vi "Brewer Palette Dialog v2.vi"() -> (0 "OK?":bool, 1 "Cancelled?":bool, 2 "Interpolate?":bool, 3 "Selected Palette Colors":u32[](array[colorbox]), 5 "Palette Name (# Colors)":string)   [LabVIEW 2021, in "Palette.lvlib"]
doc: "The Palette Colors array returned was chosen by the user while it was displayed vertically.\nIn other words, the top color is in fact color index 0, while the bottom color is in fact the last color in the array.\nTo use this array for a color ramp (or color scale), this array will need to be inverted to obtain the same visual effect."
uses:
  Palette.lvlib
  Utilities/Utilities.lvlib
  Error/Error.lvlib
  <vilib>/IlluminatedG/IG AutoComplete/AutoComplete/AutoComplete.lvlib
panel:
  in  "Matching Palette Names":i32(listbox)
  in  "Search by name":string
  in  "Show Tip Strip":bool
  out "Max  # Colors":i32=3 min=3 max=12 step=1
  in  "About":bool
  in  "Interpolate":bool
  in  "Flip Order":bool
  out "Color Ramp":dbl(ramp)
  in  "Palette List":string(combo)
  in  "Cancel":bool
  in  "OK":bool
  out "Palette Colors":u32[](array[colorbox])
  out "# Palettes":i32=3 min=3 max=12 step=1
  in  "Category":T1(ring)
  in  "photocopy safe":bool
  in  "printer friendly":bool
  in  "colorblind safe":bool
  in  "# Colors":i32=3 min=3 max=15 step=1
  in  "Background":u32(colorbox)=16777226
  # "https://colorbrewer2.org/"
  # "For a visual catalog of Brewer palettes, go to"
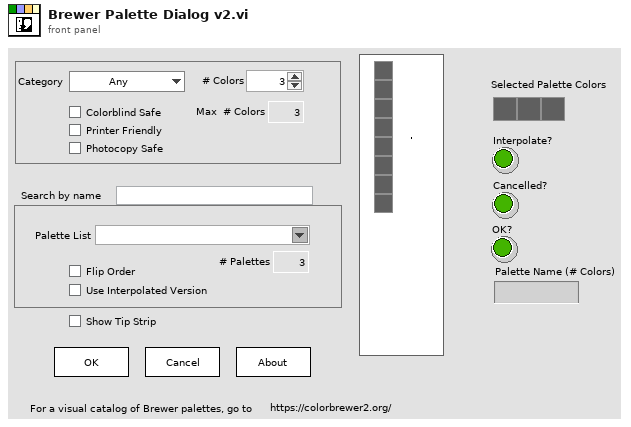
[diagram p1: front panel]
types:
  T1 = enum16{"Any", "Sequential", "Diverging", "Qualitative"}
  T2 = cluster{"Category":enum16{"Any", "Sequential", "Diverging", "Qualitative"}, "photocopy safe":bool, "printer friendly":bool, "colorblind safe":bool, "# Colors":i32, "Flip Order":bool}
  T3 = typedef "Palette.lvlib/Color Brewer Palette.ctl" = cluster{"Color Array":u32[], "Palette Name":string, "Number of Colors":i32, "Palette Category":string, "Color Blind Safe":bool, "Printer Friendly":bool, "Photocopy Safe":bool}
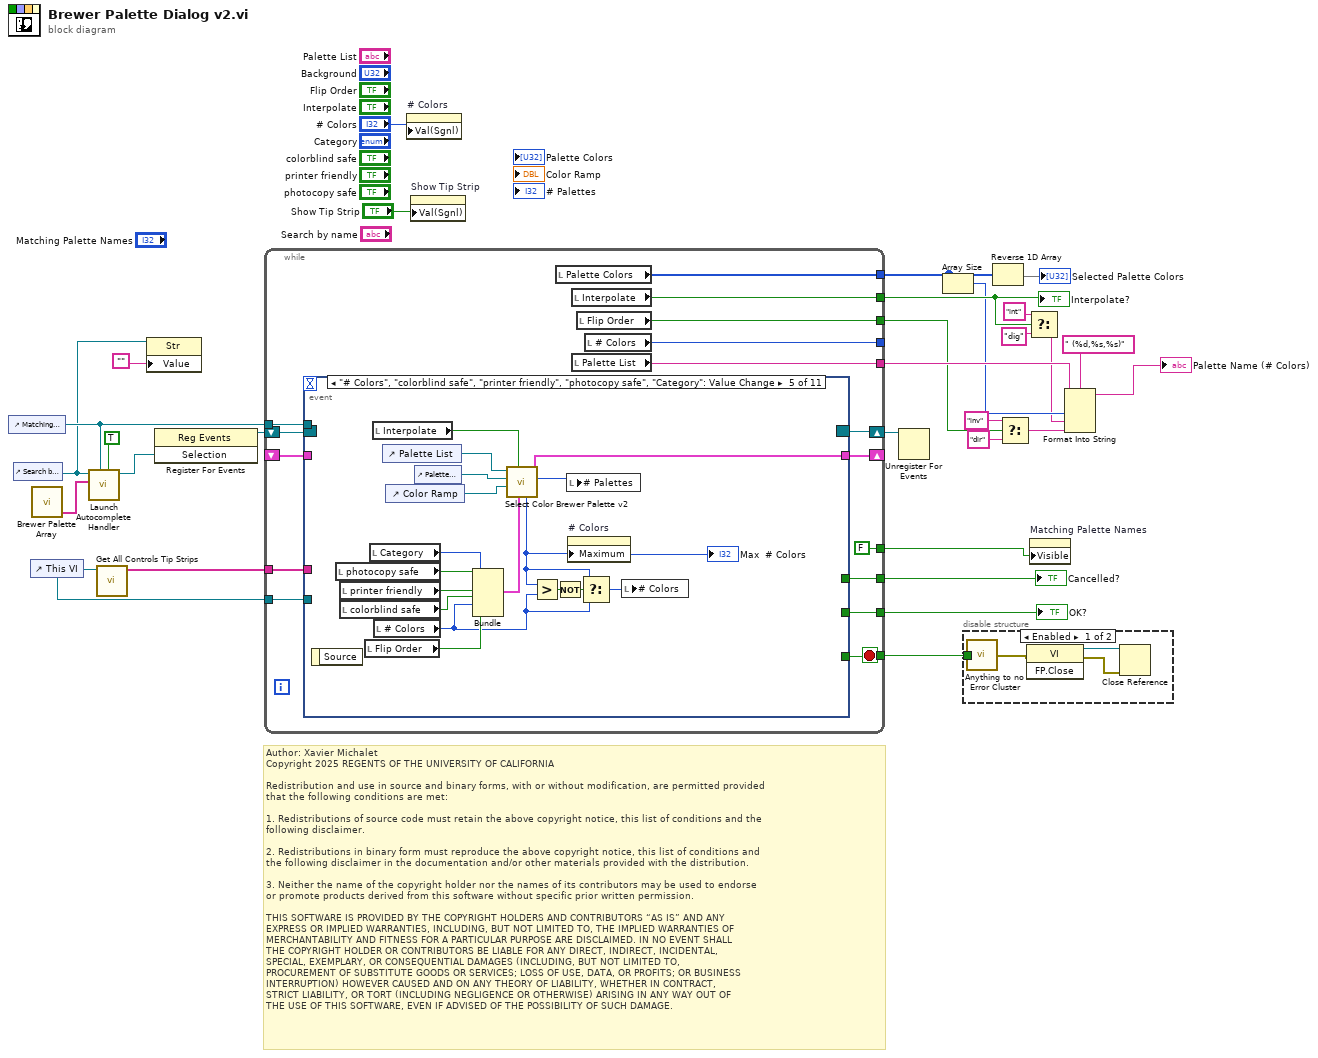
[diagram p0: block diagram]
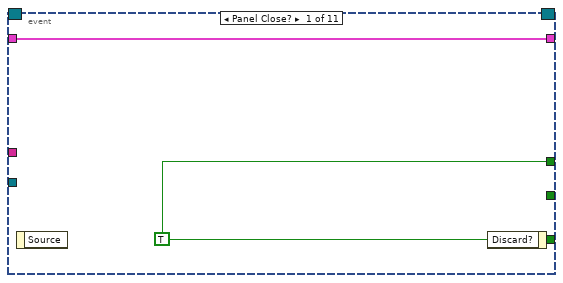
[diagram p3: hidden frame]
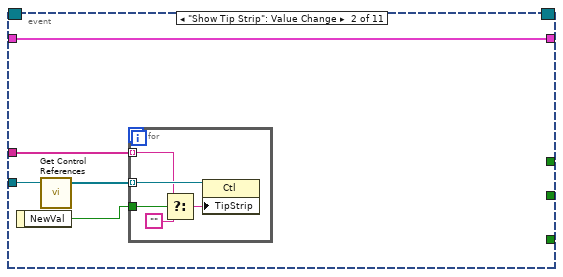
[diagram p4: hidden frame]
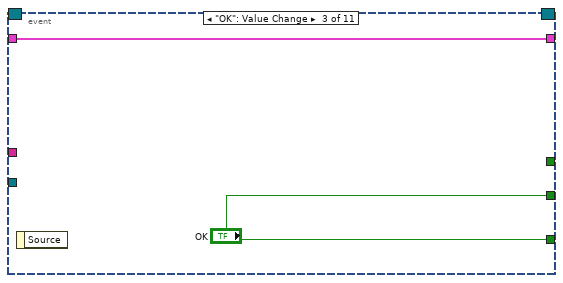
[diagram p5: hidden frame]
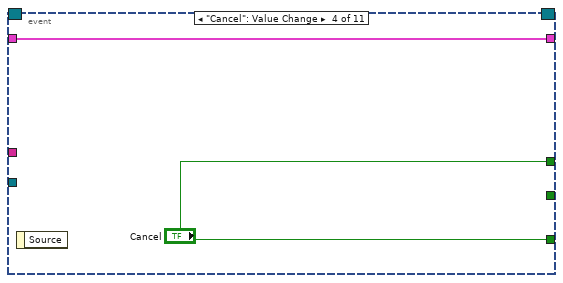
[diagram p6: hidden frame]
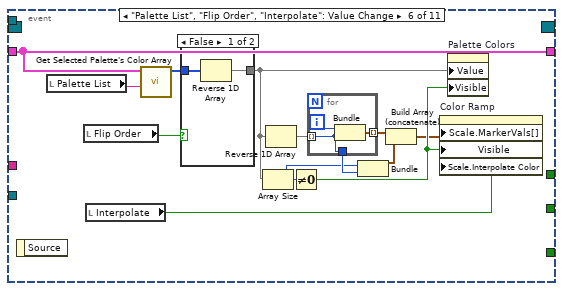
[diagram p7: hidden frame]
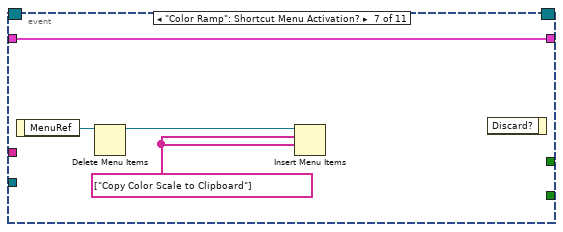
[diagram p9: hidden frame]
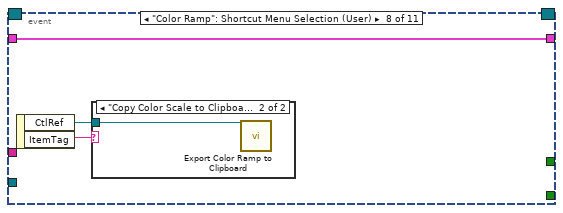
[diagram p10: hidden frame]
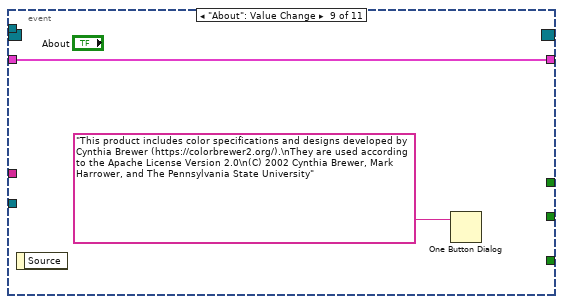
[diagram p12: hidden frame]
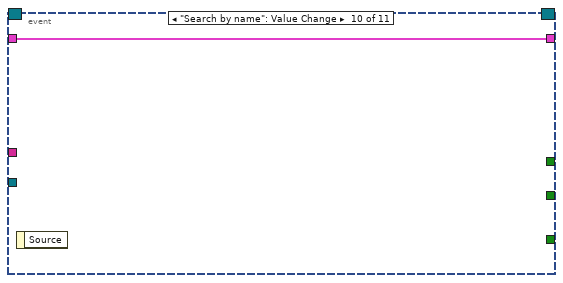
[diagram p13: hidden frame]
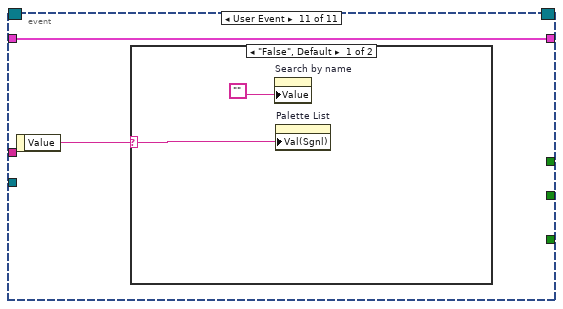
[diagram p14: hidden frame]
diagram:
  # "Author: Xavier Michalet\nCopyright 2025 REGENTS OF THE UNIVERSITY OF CALIFORNIA\n\nRedistribution and use in source and binary forms, with or without modification, are permitted provided\nthat the following conditions are met:\n\n1. Redistributions of source code must retain the above copyright notice, this list of conditions and the\nfollowing disclaimer.\n\n2. Redistributions in binary form must reproduce the above copyright notice, this list of conditions and\nthe following disclaimer in the documentation and/or other materials provided with the distribution.\n\n3. Neither the name of the copyright holder nor the names of its contributors may be used to endorse \nor promote products derived from this software without specific prior written permission.\n\nTHIS SOFTWARE IS PROVIDED BY THE COPYRIGHT HOLDERS AND CONTRIBUTORS “AS IS” AND ANY \nEXPRESS OR IMPLIED WARRANTIES, INCLUDING, BUT NOT LIMITED TO, THE IMPLIED WARRANTIES OF\nMERCHANTABILITY AND FITNESS FOR A PARTICULAR PURPOSE ARE DISCLAIMED. IN NO EVENT SHALL\nTHE COPYRIGHT HOLDER OR CONTRIBUTORS BE LIABLE FOR ANY DIRECT, INDIRECT, INCIDENTAL, \nSPECIAL, EXEMPLARY, OR CONSEQUENTIAL DAMAGES (INCLUDING, BUT NOT LIMITED TO, \nPROCUREMENT OF SUBSTITUTE GOODS OR SERVICES; LOSS OF USE, DATA, OR PROFITS; OR BUSINESS\nINTERRUPTION) HOWEVER CAUSED AND ON ANY THEORY OF LIABILITY, WHETHER IN CONTRACT, \nSTRICT LIABILITY, OR TORT (INCLUDING NEGLIGENCE OR OTHERWISE) ARISING IN ANY WAY OUT OF\nTHE USE OF THIS SOFTWARE, EVEN IF ADVISED OF THE POSSIBILITY OF SUCH DAMAGE."
  n1 = control-ref of="Matching Palette Names"() -> (w5:refnum<vi>)
  n2 = control-ref of="Search by name"() -> (w4:refnum<vi>)
  n3 = control-ref of="This VI"() -> (w11:refnum<vi>)
  n4 = call "Brewer Palette Array.vi"() -> ("Palette List"=w9:string[])  [unwired: 8 in, 1 out]
  n5 = call <vilib>:"Launch Autocomplete Handler.vi"("Autohide ListBox (F)"=TRUE, "ListBox Refnum (Popup)"=w5, "Initial Options (Empty)"=w9, "Str Refnum"=w4) -> ("Selection"=w8:refnum<user-event>)  [unwired: 4 in, 3 out]
  n6 = call "Get All Controls Tip Strips.vi"("VI Ref"=w11) -> ("Controls Tip Strips"=w13:string[])  [unwired: 9 in, 1 out]
  n7 = property class="Str"(reference=w4, "Value"="") -> ()  [unwired: 1 in, 2 out]
  n8 = register-events(w8) -> (reference out=w7:refnum<event-registration>)  [unwired: 2 in, 1 out]
  n9 = while {
    shift-right: [w46] -> _
    shift-left: _ -> [w45]
    tunnel: [w44] -> w30
    tunnel: [w43] -> w29
    tunnel: [w42] -> w27
    tunnel: [w41] -> _
    tunnel: [w40] -> w24
    tunnel: [w39] -> w22
    tunnel: [w38] -> w23
    tunnel: w11 -> [w37]
    tunnel: w13 -> [w36]
    tunnel: [w35] -> w10
    shift-right: [w33] -> w6
    shift-left: w7 -> [w34]
    tunnel: w5 -> [w32]
    tunnel: [FALSE ("Visible")] -> w1
    stop <- w35 stop-if-true
    n10 = event shown="[4] \"# Colors\", \"colorblind safe\", \"printer friendly\", \"photocopy safe\", \"Category\": Value Change" {
      selector: w34 -> [_ _ _ _ _ _ _ _ _ _ _]
      dyn-events: [_ _ _ _ _ _ _ _ _ _ _] -> w33
      timeout: _ -> [_ _ _ _ _ _ _ _ _ _ _]
      tunnel: [w47 _ "OK" "Cancel" _ _ _ _ _ _ _] -> w35
      tunnel: [w48 w53 w59 w61 w73 w92 w102 w105 w108 w109 w111] -> w46
      tunnel: w45 -> [w48 w53 w59 w61 _ w92 w102 w105 w108 w109 w111]
      tunnel: [_ _ "OK" _ _ _ _ _ _ _ _] -> w44
      tunnel: [w47 _ _ "Cancel" _ _ _ _ _ _ _] -> w43
      tunnel: w37 -> [_ w52 _ _ _ _ _ _ _ _ _]
      tunnel: w36 -> [_ w49 _ _ _ _ _ _ _ _ _]
      tunnel: w32 -> [_ _ _ _ _ _ _ _ _ _ _]
      event Panel Close? {
        w47 = TRUE ("Discard?")
        n11 = event-data() -> ()  [unwired: 1 in, 1 out]
        n12 = event-data("Discard?"=w47) -> ()  [unwired: 1 in, 1 out]
      }
      event "Show Tip Strip": Value Change {
        n13 = event-data() -> ("NewVal"=w50:bool)  [unwired: 1 in]
        n14 = call "Get Control References.vi"("VI  Ref"=w52) -> ("Controls[]"=w51:refnum<vi>[])  [unwired: 2 in, 2 out]
        n15 = for {
          tunnel: w51 -> [w58] mode=indexing
          tunnel: w50 -> [w57]
          tunnel: w49 -> [w55] mode=indexing
          n16 = Select(t=w55, s=w57, f="") -> (s? t:f=w56:string)
          n17 = property class="Ctl"(reference=w58, "TipStrip"=w56) -> ()  [unwired: 1 in, 2 out]
        }
      }
      event "OK": Value Change {
        n18 = event-data() -> ()  [unwired: 1 in, 1 out]
      }
      event "Cancel": Value Change {
        n19 = event-data() -> ()  [unwired: 1 in, 1 out]
      }
      event "# Colors", "colorblind safe", "printer friendly", "photocopy safe", "Category": Value Change {
        n20 = event-data() -> ()  [unwired: 1 in, 1 out]
        n21 = local read "photocopy safe"() -> (w78:bool)
        n22 = local read "printer friendly"() -> (w77:bool)
        n23 = local read "colorblind safe"() -> (w76:bool)
        n24 = local read "Flip Order"() -> (w69:bool)
        n25 = local read "Category"() -> (w79:T1)
        n26 = local read "Interpolate"() -> (w63:bool)
        n27 = local read "# Colors"() -> (w67:i32)
        n28 = control-ref of="Palette List"() -> (w72:refnum<vi>)
        n29 = control-ref of="Color Ramp"() -> (w70:refnum<vi>)
        n30 = control-ref of="Palette Colors"() -> (w75:refnum<vi>)
        n31 = Bundle("Category"=w79, "photocopy safe"=w78, "printer friendly"=w77, "colorblind safe"=w76, "# Colors"=w67, "Flip Order"=w69) -> (w71:T2)  [unwired: 1 in]
        n32 = call "Select Color Brewer Palette v2.vi"("User Choices"=w71, "Interpolate"=w63, "Color Ramp Refnum"=w70, "Palette Colors"=w75, "Palette List Refnum"=w72) -> ("# Palettes"=w74:i32, "Available Palettes"=w73:T3[], "Compatible Max # Colors"=w64:i32)  [unwired: 2 in, 2 out]
        "Max  # Colors" <- w64
        n33 = Greater?(x=w64, y=w67) -> (0:w68:bool)
        n34 = Not(x=w68) -> (.not. x?=w65:bool)
        n35 = local write "# Palettes"(w74) -> ()
        n36 = property on="# Colors" class="DigNum (strict)"("Maximum"=w64) -> ()  [unwired: 2 in, 2 out]
        n37 = Select(t=w64, s=w65, f=w67) -> (s? t:f=w66:i32)
        n38 = local write "# Colors"(w66) -> ()
      }
      event "Palette List", "Flip Order", "Interpolate": Value Change {
        n39 = event-data() -> ()  [unwired: 1 in, 1 out]
        n40 = local read "Palette List"() -> (w87:string)
        n41 = local read "Flip Order"() -> (w91:bool)
        n42 = local read "Interpolate"() -> (w84:bool)
        n43 = call "Get Selected Palette's Color Array.vi"("Selected Palette"=w87, "Palette Specifications"=w92) -> ("Palette Colors"=w90:u32[])  [unwired: 8 in, 1 out]
        n44 = case shown="False" w91 {
          tunnel: w90 -> [w97 w98]
          tunnel: [w96 w98] -> w86
          frame False {
            n45 = Reverse 1D Array(array=w97) -> (reversed array=w96:u32[])
          }
          frame True {
          }
        }
        n46 = Array Size(array=w86) -> (size(s)=w80:i32)
        n47 = Reverse 1D Array(array=w86) -> (reversed array=w89:u32[])
        n48 = Not Equal To 0?(x=w80) -> (x != 0?=w85:bool)
        n49 = for {
          tunnel: w89 -> [w93] mode=indexing
          tunnel: [w94] -> w88 mode=indexing
          tunnel: [w93] -> w81
          i -> [w95]
          n50 = Bundle(w95, "Color Box"=w93) -> (w94:cluster{i32, "Color Box":u32})  [unwired: 1 in]
        }
        n51 = Bundle(w80, "Color Box"=w81) -> (w82:cluster{i32, "Color Box":u32})  [unwired: 1 in]
        n52 = Build Array (concatenate)(w88, w82) -> (w83:cluster{i32, "Color Box":u32}[])
        n53 = property on="Color Ramp" class="ColRmp (strict)"("Scale.MarkerVals[]"=w83, "Visible"=w85, "Scale.Interpolate Color"=w84) -> ()  [unwired: 2 in, 2 out]
        n54 = property on="Palette Colors" class="Arr (strict)"("Value"=w86, "Visible"=w85) -> ()  [unwired: 2 in, 2 out]
      }
      event "Color Ramp": Shortcut Menu Activation? {
        w100 = string[] ["Copy Color Scale to Clipboard"] ("item names")
        n55 = event-data() -> ("MenuRef"=w99:refnum<k9>)  [unwired: 1 in]
        n56 = Delete Menu Items(9:w99) -> (3:w101:refnum<k9>)  [unwired: 3 in, 1 out]
        n57 = Insert Menu Items(7:w100, 8:w100, 9:w101) -> ()  [unwired: 3 in, 3 out]
        n58 = event-data() -> ()  [unwired: 2 in, 1 out]
      }
      event "Color Ramp": Shortcut Menu Selection (User) {
        n59 = event-data() -> ("CtlRef"=w103:refnum<vi>, "ItemTag"=w104:string)  [unwired: 1 in]
        n60 = case shown="\"Copy Color Scale to Clipboard\"" w104 {
          tunnel: w103 -> [_ w106]
          frame "", Default {
          }
          frame "Copy Color Scale to Clipboard" {
            n61 = call "Export Color Ramp to Clipboard.vi"("ColorRamp in"=w106) -> ()  [unwired: 11 in]
          }
        }
      }
      event "About": Value Change {
        n62 = event-data() -> ()  [unwired: 1 in, 1 out]
        n63 = One Button Dialog(message="This product includes color specifications and designs developed by Cynthia Brewer (https://colorbrewer2.org/).\nThey are used according to the Apache License Version 2.0\n(C) 2002 Cynthia Brewer, Mark Harrower, and The Pennsylvania State University" ("Text")) -> ()  [unwired: 1 in, 1 out]
      }
      event "Search by name": Value Change {
        n64 = event-data() -> ()  [unwired: 1 in, 1 out]
      }
      event User Event {
        n65 = event-data() -> ("Value"=w110:string)  [unwired: 1 in]
        n66 = case shown="\"False\", Default" w110 {
          selector: w110 -> [w113 _]
          frame "False", Default {
            n67 = property on="Search by name" class="Str"("Value"="") -> ()  [unwired: 2 in, 2 out]
            n68 = property on="Palette List" class="CmbBox"("Val(Sgnl)"=w113) -> ()  [unwired: 2 in, 2 out]
          }
          frame "" {
          }
        }
      }
    }
    n69 = local read "Palette Colors"() -> (w39:u32[])
    n70 = local read "Interpolate"() -> (w40:bool)
    n71 = local read "Palette List"() -> (w42:string)
    n72 = local read "Flip Order"() -> (w38:bool)
    n73 = local read "# Colors"() -> (w41:i32)
  }
  "OK?" <- w30
  "Cancelled?" <- w29
  "Interpolate?" <- w24
  n74 = property on="# Colors" class="DigNum (strict)"("Val(Sgnl)"="# Colors") -> ()  [unwired: 2 in, 2 out]
  n75 = property on="Show Tip Strip" class="Bool (strict)"("Val(Sgnl)"="Show Tip Strip") -> ()  [unwired: 2 in, 2 out]
  n76 = Unregister For Events(event registration refnum=w6) -> ()  [unwired: 1 in, 1 out]
  n77 = Array Size(array=w22) -> (size(s)=w21:i32)
  n78 = disable-structure shown="Enabled" {
    disable-tunnel: w10 -> [w115 _]
    frame Enabled {
      n79 = call "Anything to no Error Cluster.vi"("Variant"=w115) -> ("Error Out"=w114:errorcluster)  [unwired: 8 in]
      n80 = invoke class="VI" method="FP.Close"(error in=w114) -> (reference out=w117:refnum<vi>, error out=w116:errorcluster)  [unwired: 2 in, 1 out]
      n81 = Close Reference(reference=w117, error in (no error)=w116) -> ()  [unwired: 1 out]
    }
    frame Disabled {
    }
  }
  n82 = Reverse 1D Array(array=w22) -> (reversed array=→"Selected Palette Colors":u32[])
  n83 = Select(t="inv" ("input 2"), s=w23, f="dir") -> (s? t:f=w15:string)
  n84 = Select(t="int" ("input 2"), s=w24, f="dig") -> (s? t:f=w17:string)
  n85 = property on="Matching Palette Names" class="LstBox (strict)"("Visible"=w1) -> ()  [unwired: 2 in, 2 out]
  n86 = Format Into String(format string=" (%d,%s,%s)", initial string=w27, w21, w17, w15) -> (resulting string=→"Palette Name (# Colors)":string)  [unwired: 1 in, 1 out]
